vi "Test Deserialize Timestamps.vi"(8 "error in (no error)":errorcluster) -> (0 "error out":errorcluster)   [LabVIEW 2013]
uses:
  src/Serializer/JSON Serializer/JSON Serializer.lvclass
  src/Deserializer/JSON Deserializer/JSON Deserializer.lvclass
  <vilib>/addons/_JKI Toolkits/Caraya/classes/Test/Test.lvclass
  <vilib>/addons/_JKI Toolkits/Caraya/classes/Assert/Assert.lvclass
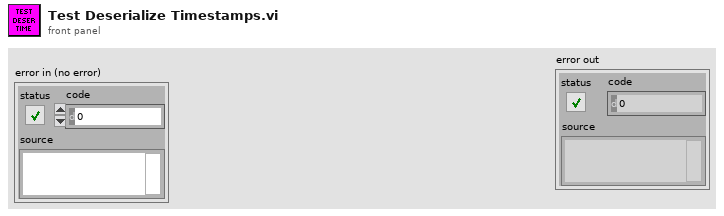
[diagram p1: front panel]
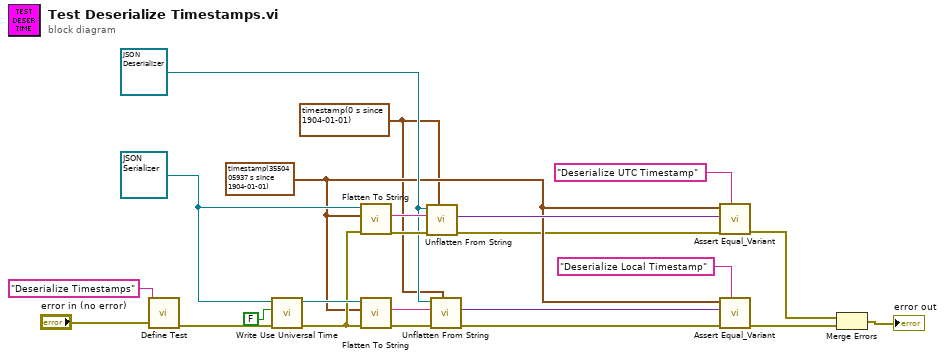
[diagram p0: block diagram]
diagram:
  w1 = timestamp(0 s since 1904-01-01)
  w8 = refnum<class "JSON Deserializer.lvclass"> refnum ("Deserializer in")
  w5 = timestamp(3550405937.679 s since 1904-01-01)
  w16 = refnum<class "JSON Serializer.lvclass"> refnum ("JKI JSON Serialization.lvlib:JSON Serializer.lvclass")
  n1 = call <vilib>:"Define Test.vi"("error in (no error)"="error in (no error)", "Label (VI Title)"="Deserialize Timestamps") -> ("error out"=w14:errorcluster)  [unwired: 9 in]
  n2 = call-dynamic "Write Use Universal Time.vi"("error in (no error)"=w14, "Universal Time"=FALSE, "JSON Serializer in"=w16) -> ("error out"=w13:errorcluster, "JSON Serializer out"=w15:refnum<class "JSON Serializer.lvclass">)  [unwired: 7 in]
  n3 = call-dynamic "Flatten To String.vi"("error in (no error)"=w13, "Variant"=w5, "JSON Serializer in"=w16) -> ("error out"=w10:errorcluster, "String"=w11:string)  [unwired: 6 in, 1 out]
  n4 = call-dynamic "Flatten To String.vi"("error in (no error)"=w13, "Variant"=w5, "JSON Serializer in"=w15) -> ("error out"=w9:errorcluster, "String"=w7:string)  [unwired: 6 in, 1 out]
  n5 = call-dynamic "Unflatten From String.vi"("Type and Defaults"=w1, "error in (no error)"=w10, "String"=w11, "Deserializer in"=w8) -> ("error out"=w2:errorcluster, "Variant"=w6:variant)  [unwired: 5 in, 1 out]
  n6 = call-dynamic "Unflatten From String.vi"("Type and Defaults"=w1, "error in (no error)"=w9, "String"=w7, "Deserializer in"=w8) -> ("error out"=w3:errorcluster, "Variant"=w4:variant)  [unwired: 5 in, 1 out]
  n7 = call <vilib>:"Assert Equal_Variant.vi"("Label"="Deserialize UTC Timestamp", "error in (no error)"=w2, "Y"=w6, "X"=w5) -> ("error out"=w18:errorcluster)  [unwired: 7 in]
  n8 = call <vilib>:"Assert Equal_Variant.vi"("Label"="Deserialize Local Timestamp", "error in (no error)"=w3, "Y"=w4, "X"=w5) -> ("error out"=w19:errorcluster)  [unwired: 7 in]
  n9 = Merge Errors(w18, w19) -> (→"error out":errorcluster)
